vi "TEST_ActorFramework.vi"() -> (0 "error description out":T2)   [LabVIEW 2024]
uses:
  utility.llb/error type.ctl
  utility.llb/error description.ctl
  utility.llb/array of error description.ctl
  Messaging Tests.lvclass
  <vilib>/ActorFramework/Time-Delayed Send Message/Time-Delay Override Options.ctl
panel:
  in  "Name Ring":T1(ring)
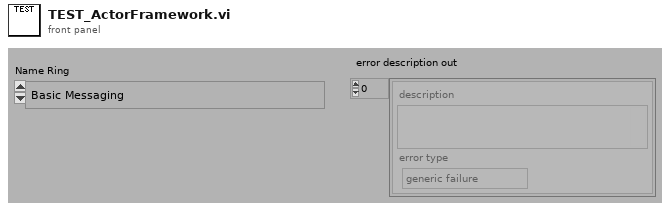
[diagram p1: front panel]
types:
  T1 = enum32{"Basic Messaging", "Priority Queue Test", "Self Messaging", "Batch Messaging", "Reply Messaging", "Timed Messaging_Stop All Further", "Timed Messaging_Send Next Then Stop", "Timed Messaging_Skip Next", "Timed Messaging_Send Next Now", "Pre-Launch Init Error"}
  T2 = typedef "array of error description.ctl" = T3[]
  T3 = typedef "error description.ctl" = cluster{"description":string, "error type":T4}
  T4 = typedef "error type.ctl" = enum32{"generic failure", "boundary case", "precision", "expected error"}
  T5 = typedef "Time-Delay Override Options.ctl" = enum16{"Send next copy now", "Skip next scheduled copy", "Send next copy now and stop all further copies", "Stop all further copies"}
  T6 = enum32{"invalid app kind", "Development System", "Run Time System", "Student Edition", "Embedded LabVIEW", "Evaluation", "Custom"}
  T7 = enum16{"open", "replace", "create", "open or create", "replace or create", "replace or create with confirmation"}
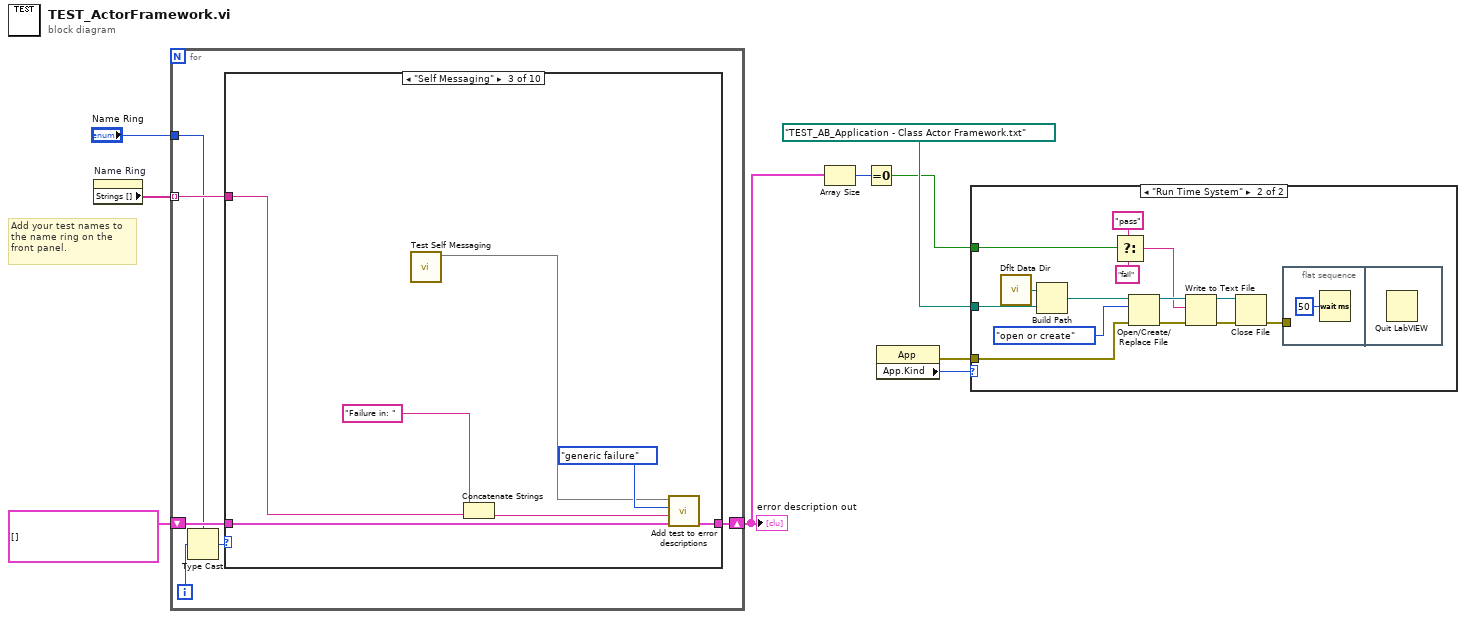
[diagram p0: block diagram]
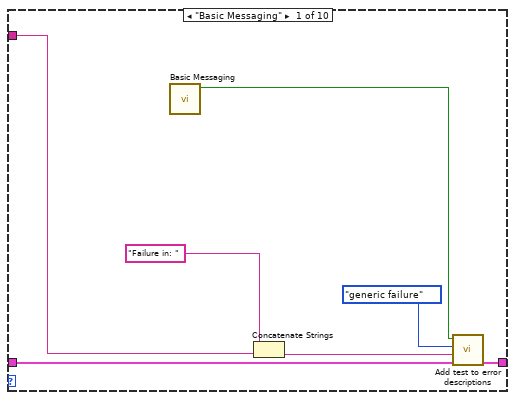
[diagram p3: hidden frame]
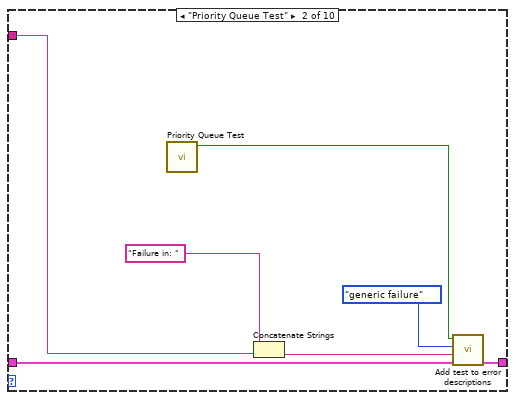
[diagram p4: hidden frame]
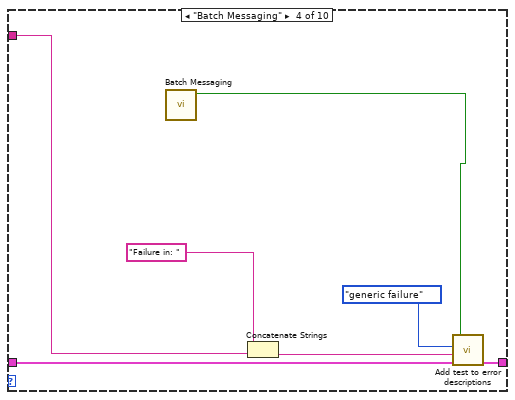
[diagram p5: hidden frame]
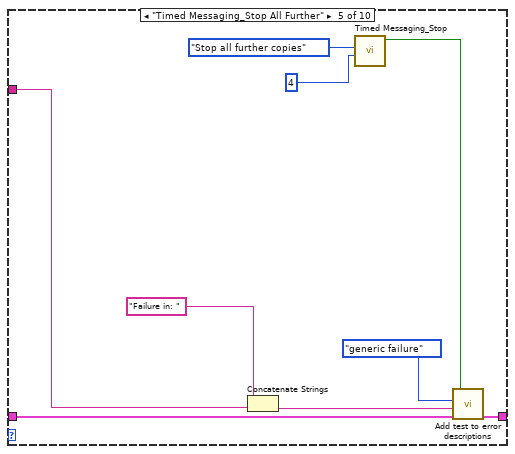
[diagram p6: hidden frame]
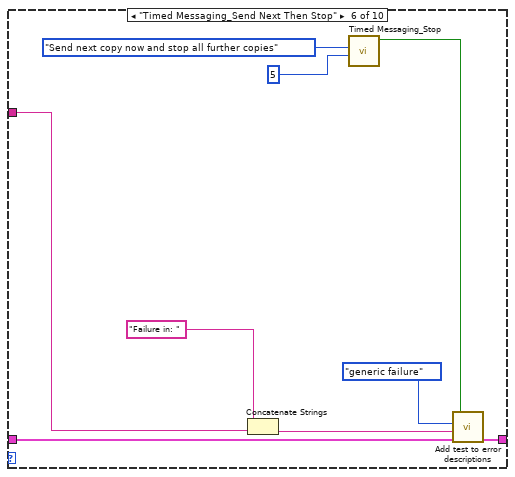
[diagram p7: hidden frame]
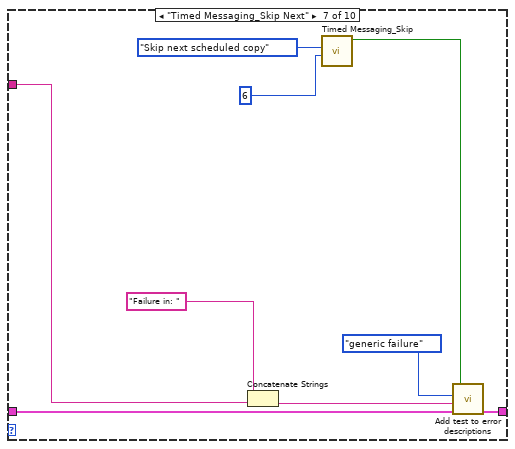
[diagram p8: hidden frame]
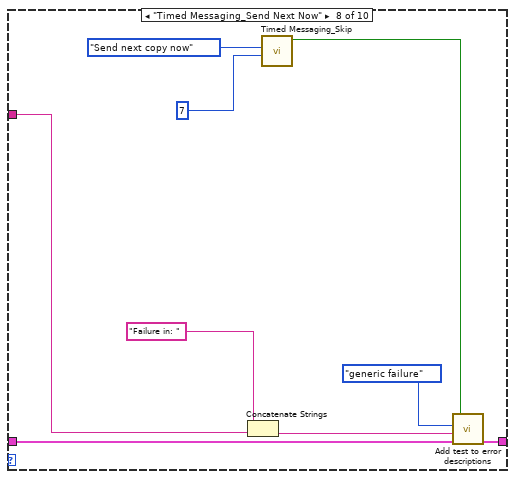
[diagram p9: hidden frame]
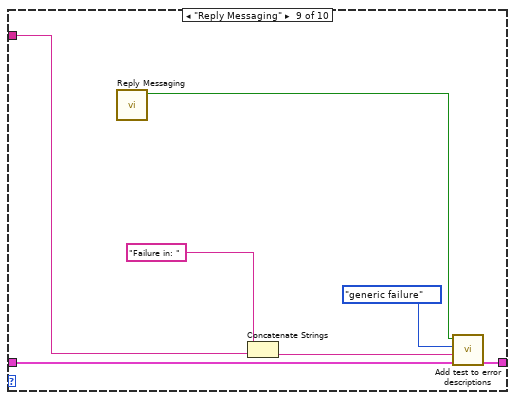
[diagram p10: hidden frame]
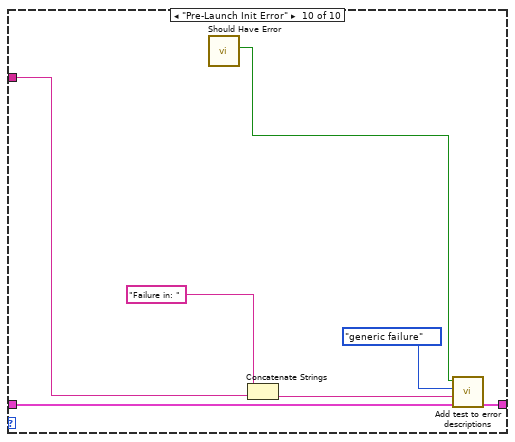
[diagram p11: hidden frame]
diagram:
  # "Add your test names to \nthe name ring on the \nfront panel."
  n1 = property on="Name Ring" class="Enum (strict)"() -> ("Strings []"=w8:string[])  [unwired: 2 in, 2 out]
  n2 = for {
    shift-right: [w15] -> w3
    shift-left: T2 [] ("error descriptions in") -> [w14]
    tunnel: w8 -> [w12] mode=indexing
    tunnel: "Name Ring" -> [w11]
    i -> [w10]
    n3 = Type Cast(type=w11, x=w10) -> (*(type *) &x=w13:T1)
    n4 = case shown="\"Self Messaging\"" w13 {
      tunnel: [w22 w29 w36 w43 w52 w61 w70 w79 w86 w93] -> w15
      tunnel: w14 -> [w21 w28 w35 w42 w51 w60 w69 w78 w85 w92]
      tunnel: w12 -> [w18 w25 w31 w38 w47 w56 w65 w74 w81 w88]
      frame "Basic Messaging" {
        n5 = call "Basic Messaging.vi"() -> ("Pass?"=w16:bool)  [unwired: 11 in]
        n6 = Concatenate Strings("Failure in: " ("error string"), w18) -> (w17:string)
        n7 = call "Add test to error descriptions.vi"("error descriptions in"=w21, "error string"=w17, "error type"=error_type."generic failure", "pass"=w16) -> ("error description out"=w22:T2)  [unwired: 3 in]
      }
      frame "Priority Queue Test" {
        n8 = call "Priority Queue Test.vi"() -> ("Pass?"=w23:bool)  [unwired: 11 in]
        n9 = Concatenate Strings("Failure in: " ("error string"), w25) -> (w24:string)
        n10 = call "Add test to error descriptions.vi"("error descriptions in"=w28, "error string"=w24, "error type"=error_type."generic failure", "pass"=w23) -> ("error description out"=w29:T2)  [unwired: 3 in]
      }
      frame "Self Messaging" {
        n11 = call "Test Self Messaging.vi"() -> (3:w30)  [unwired: 11 in]
        n12 = Concatenate Strings("Failure in: " ("error string"), w31) -> (w32:string)
        n13 = call "Add test to error descriptions.vi"("error descriptions in"=w35, "error string"=w32, "error type"=error_type."generic failure", "pass"=w30) -> ("error description out"=w36:T2)  [unwired: 3 in]
      }
      frame "Batch Messaging" {
        n14 = call "Batch Messaging.vi"() -> ("Pass?"=w37:bool)  [unwired: 11 in]
        n15 = Concatenate Strings("Failure in: " ("error string"), w38) -> (w39:string)
        n16 = call "Add test to error descriptions.vi"("error descriptions in"=w42, "error string"=w39, "error type"=error_type."generic failure", "pass"=w37) -> ("error description out"=w43:T2)  [unwired: 3 in]
      }
      frame "Timed Messaging_Stop All Further" {
        n17 = Concatenate Strings("Failure in: " ("error string"), w47) -> (w48:string)
        n18 = call "Timed Messaging_Stop.vi"("expected"=4, "notification"=Time-Delay_Override_Options."Stop all further copies") -> ("Pass?"=w46:bool)  [unwired: 9 in]
        n19 = call "Add test to error descriptions.vi"("error descriptions in"=w51, "error string"=w48, "error type"=error_type."generic failure", "pass"=w46) -> ("error description out"=w52:T2)  [unwired: 3 in]
      }
      frame "Timed Messaging_Send Next Then Stop" {
        n20 = Concatenate Strings("Failure in: " ("error string"), w56) -> (w57:string)
        n21 = call "Timed Messaging_Stop.vi"("expected"=5, "notification"=Time-Delay_Override_Options."Send next copy now and stop all further copies") -> ("Pass?"=w55:bool)  [unwired: 9 in]
        n22 = call "Add test to error descriptions.vi"("error descriptions in"=w60, "error string"=w57, "error type"=error_type."generic failure", "pass"=w55) -> ("error description out"=w61:T2)  [unwired: 3 in]
      }
      frame "Timed Messaging_Skip Next" {
        n23 = Concatenate Strings("Failure in: " ("error string"), w65) -> (w66:string)
        n24 = call "Timed Messaging_Skip.vi"("expected"=6, "notification"=Time-Delay_Override_Options."Skip next scheduled copy") -> ("Pass?"=w64:bool)  [unwired: 9 in]
        n25 = call "Add test to error descriptions.vi"("error descriptions in"=w69, "error string"=w66, "error type"=error_type."generic failure", "pass"=w64) -> ("error description out"=w70:T2)  [unwired: 3 in]
      }
      frame "Timed Messaging_Send Next Now" {
        n26 = Concatenate Strings("Failure in: " ("error string"), w74) -> (w75:string)
        n27 = call "Timed Messaging_Skip.vi"("expected"=7, "notification"=Time-Delay_Override_Options."Send next copy now") -> ("Pass?"=w73:bool)  [unwired: 9 in]
        n28 = call "Add test to error descriptions.vi"("error descriptions in"=w78, "error string"=w75, "error type"=error_type."generic failure", "pass"=w73) -> ("error description out"=w79:T2)  [unwired: 3 in]
      }
      frame "Reply Messaging" {
        n29 = call "Reply Messaging.vi"() -> ("Pass?"=w80:bool)  [unwired: 11 in]
        n30 = Concatenate Strings("Failure in: " ("error string"), w81) -> (w82:string)
        n31 = call "Add test to error descriptions.vi"("error descriptions in"=w85, "error string"=w82, "error type"=error_type."generic failure", "pass"=w80) -> ("error description out"=w86:T2)  [unwired: 3 in]
      }
      frame "Pre-Launch Init Error" {
        n32 = call "Should Have Error.vi"() -> ("Pass?"=w87:bool)  [unwired: 11 in]
        n33 = Concatenate Strings("Failure in: " ("error string"), w88) -> (w89:string)
        n34 = call "Add test to error descriptions.vi"("error descriptions in"=w92, "error string"=w89, "error type"=error_type."generic failure", "pass"=w87) -> ("error description out"=w93:T2)  [unwired: 3 in]
      }
    }
  }
  "error description out" <- w3
  n35 = Array Size(array=w3) -> (size(s)=w2:i32)
  n36 = Equal To 0?(x=w2) -> (x = 0?=w1:bool)
  n37 = property class="App"() -> (error out=w4:errorcluster, "App.Kind"=w6:T6)  [unwired: 2 in, 1 out]
  n38 = case shown="\"Run Time System\"" w6 {
    tunnel: path "TEST_AB_Application - Class Actor Framework.txt" -> [_ w96]
    tunnel: w4 -> [_ w95]
    tunnel: w1 -> [_ w94]
    frame Default {
    }
    frame "Run Time System" {
      n39 = call <vilib>:"Dflt Data Dir.vi"() -> ("App:Default Data Directory"=w99:path)
      n40 = Build Path(base path=w99, name or relative path=w96) -> (appended path=w98:path)
      n41 = Select(t="pass" ("name or relative path"), s=w94, f="fail" ("name or relative path")) -> (s? t:f=w100:string)
      n42 = Open/Create/Replace File(file path (use dialog)=w98, error in=w95, operation (0:open)=T7."open or create") -> (refnum out=w107:refnum<file>, error out=w106:errorcluster)  [unwired: 3 in, 1 out]
      n43 = Write to Text File(file (use dialog)=w107, text=w100, error in=w106) -> (refnum out=w103:refnum<file>, error out=w104:errorcluster)  [unwired: 1 in, 1 out]
      n44 = Close File(refnum=w103, error in=w104) -> (error out=w97:errorcluster)  [unwired: 1 out]
      n45 = flat-sequence {
        tunnel: w97 -> [_]
        frame #0 {
          n46 = Wait (ms)(milliseconds to wait=u32 50) -> ()  [unwired: 1 out]
        }
        frame #1 {
          n47 = Quit LabVIEW() -> ()  [unwired: 1 in]
        }
      }
    }
  }
